vi "Load TS Configuration.vi"(8 "error in":errorcluster, 10 "Config File refnum in":T1, 11 "Generic Test Stand in":refnum<class "Generic Test Stand.lvclass">) -> (0 "error out":errorcluster, 2 "Config File refnum out":T1, 3 "Generic Test Stand out":refnum<class "Generic Test Stand.lvclass">)   [LabVIEW 2019, in "Generic Test Stand.lvclass"]
uses:
  Generic Test Stand.lvclass
  <vilib>/Utility/config.llb/Config Data RefNum.ctl
  Generic Test Stand.lvclass/Generic Test Stand.ctl
  <vilib>/Utility/config.llb/Read Key (U32).vi
  <vilib>/Utility/config.llb/Read Key (String).vi
  <vilib>/Utility/config.llb/NI_LVConfig.lvlib
  <vilib>/Utility/config.llb/Read Key (Double).vi
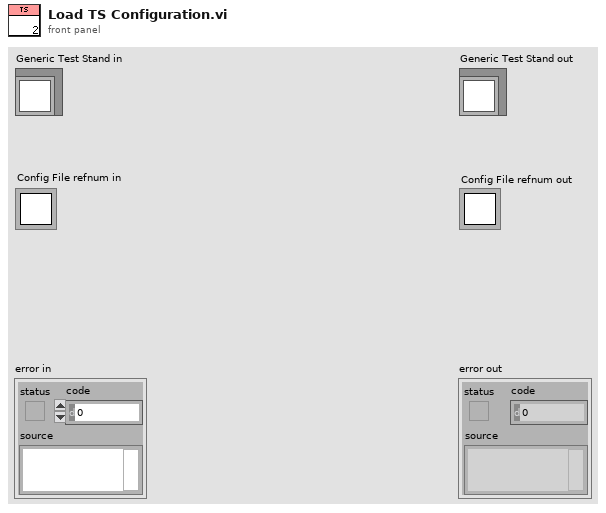
[diagram p1: front panel]
types:
  T1 = typedef "NI_LVConfig.lvlib/Config Data RefNum.ctl" = refnum<k1>
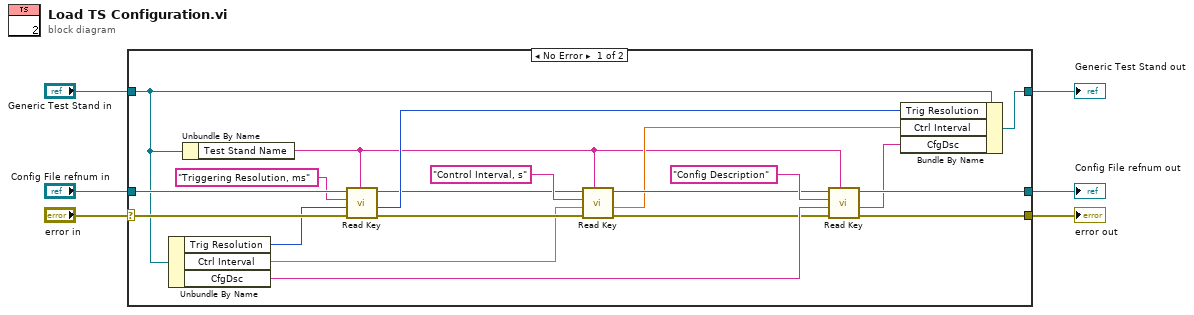
[diagram p0: block diagram]
diagram:
  n1 = case shown="No Error" "error in" {
    selector: "error in" -> [w24 w29]
    tunnel: [w21 w29] -> w5
    tunnel: [w23 w28] -> w3
    tunnel: "Generic Test Stand in" -> [w18 w28]
    tunnel: "Config File refnum in" -> [w26 w27]
    tunnel: [w22 w27] -> w1
    frame No Error {
      n2 = Unbundle By Name(w18) -> ("Trig Resolution"=w16:u32, "Ctrl Interval"=w9:dbl, "CfgDsc"=w17:string)
      n3 = Unbundle By Name(w18) -> ("Test Stand Name"=w7:string)
      n4 = call-poly <vilib>:"Read Key.vi"("section"=w7, "error in (no error)"=w24, "default value"=w16, "key"="Triggering Resolution, ms", "refnum"=w26) -> ("error out"=w13:errorcluster, "value"=w15:u32, "refnum out"=w11:T1)  [unwired: 3 in, 1 out]
      n5 = call-poly <vilib>:"Read Key.vi"("section"=w7, "error in (no error)"=w13, "default value"=w9, "key"="Control Interval, s", "refnum"=w11) -> ("error out"=w12:errorcluster, "value"=w8:dbl, "refnum out"=w10:T1)  [unwired: 3 in, 1 out]
      n6 = call-poly <vilib>:"Read Key.vi"("section"=w7, "error in (no error)"=w12, "default value"=w17, "key"="Config Description", "refnum"=w10) -> ("error out"=w21:errorcluster, "value"=w19:string, "refnum out"=w22:T1)  [unwired: 3 in, 1 out]
      n7 = Bundle By Name(cluster=w18, "Trig Resolution"=w15, "Ctrl Interval"=w8, "CfgDsc"=w19) -> (w23:refnum<class "Generic Test Stand.lvclass">)
    }
    frame Error {
    }
  }
  "error out" <- w5
  "Generic Test Stand out" <- w3
  "Config File refnum out" <- w1
